vi "InitializeBkPrecision.vi"(0 "COM Port":refnum<visa-resource-name>) -> (1 "error out":errorcluster, 2 "VISA resource name out":refnum<visa-resource-name>)   [LabVIEW 2010]
uses:
  <instrlib>/BK Precision 85XX Series/BK Precision 85XX Series.lvlib
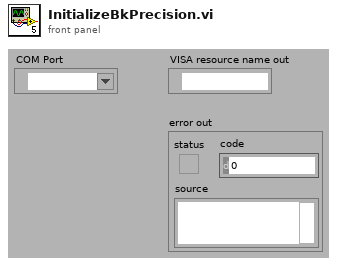
[diagram p1: front panel]
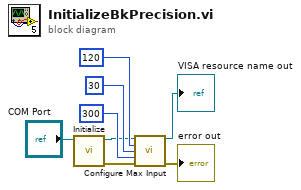
[diagram p0: block diagram]
diagram:
  n1 = call <instrlib>:"Initialize.vi"("VISA resource name"="COM Port") -> ("error out"=w3:errorcluster, "VISA resource name out"=w2:refnum<visa-resource-name>)  [unwired: 9 in]
  n2 = call <instrlib>:"Configure Max Input.vi"("VISA resource name"=w2, "Maximum Input Voltage (0)"=120, "Maximum Input Current (0)"=30, "Maximum Input Power (0)"=300, "error in (no error)"=w3) -> ("VISA resource name out"=→"VISA resource name out":refnum<visa-resource-name>, "error out"=→"error out":errorcluster)  [unwired: 9 in]
